vi "Execute Default event.vi"(4 "Module type":T1, 6 "Module ID":i32, 8 "error in":errorcluster, 9 "Event":string, 10 "DQMH Library Ref":refnum<vi>, 11 "application Instance":refnum<vi>) -> (0 "error out":errorcluster)   [LabVIEW 2019, in "Panther Dashboard.lvlib"]
doc: "This VI checks the Main.vi State of the selected DQMH Module"
uses:
  Panther Dashboard.lvlib
  Module type--enum.ctl
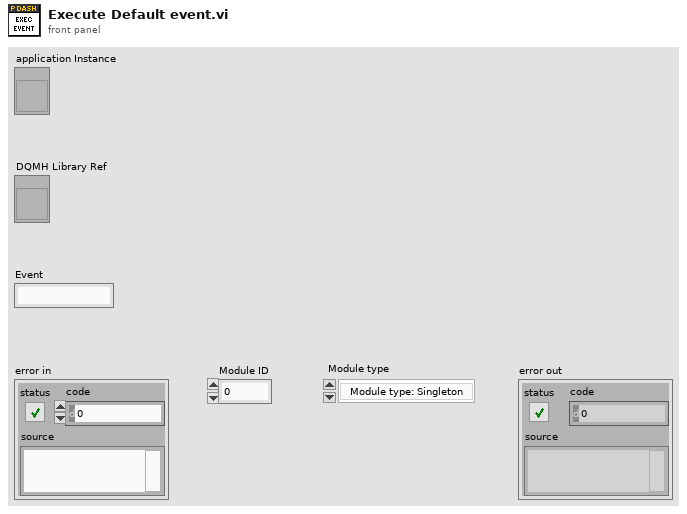
[diagram p1: front panel]
types:
  T1 = typedef "Panther Dashboard.lvlib/Module type--enum.ctl" = enum16{"Module type: Singleton", "Module type: Cloneable"}
  T2 = enum32{"Bad", "Idle", "Run top level", "Running"}
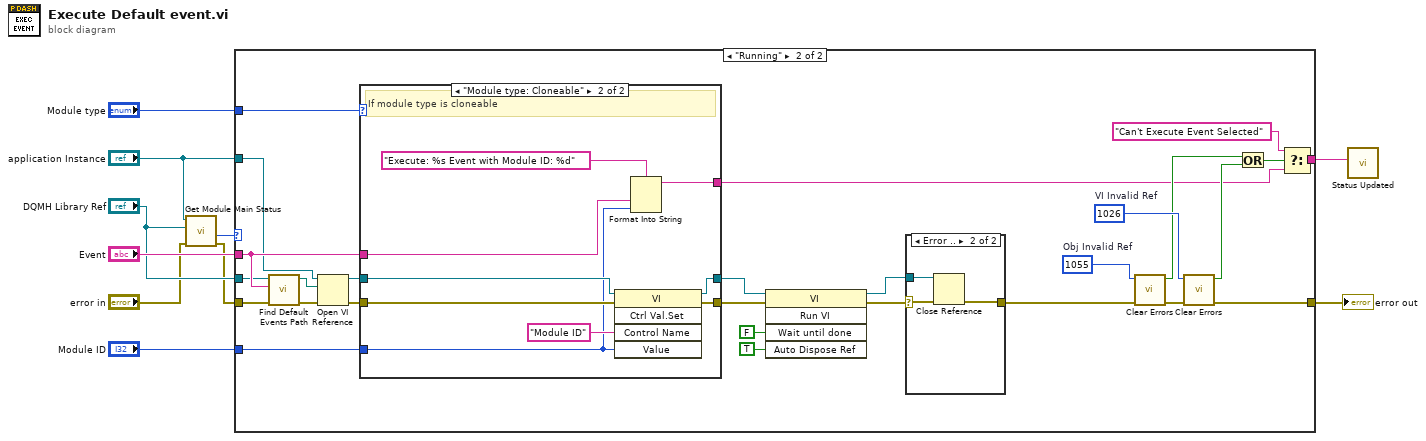
[diagram p0: block diagram]
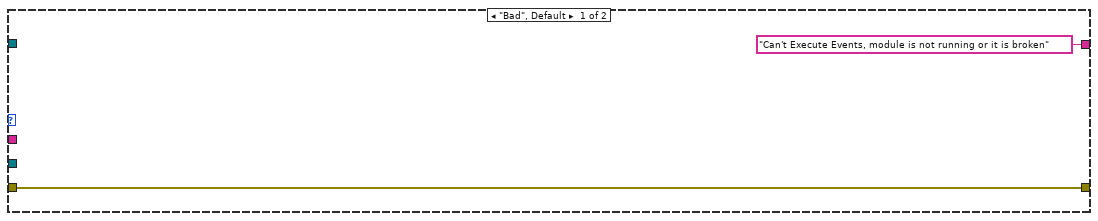
[diagram p2: hidden frame]
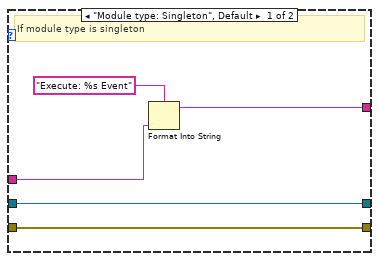
[diagram p4: hidden frame]
diagram:
  n1 = call "Get Module Main Status.vi"("error in"="error in", "Library in"="DQMH Library Ref", "application Instance"="application Instance") -> ("error out"=w1:errorcluster, "Module Exec State"=w3:T2)  [unwired: 6 in, 1 out]
  n2 = case shown="\"Running\"" w3 {
    tunnel: w1 -> [w12 w39]
    tunnel: [w12 w36] -> w10
    tunnel: "Module type" -> [_ w28]
    tunnel: "Module ID" -> [_ w26]
    tunnel: "Event" -> [_ w22]
    tunnel: ["Can't Execute Events, module is not running or it is broken" ("t") w17] -> w6
    tunnel: "application Instance" -> [_ w14]
    tunnel: "DQMH Library Ref" -> [_ w13]
    frame "Bad", Default {
    }
    frame "Running" {
      w30 = 1055  # Obj Invalid Ref
      w29 = 1026  # VI Invalid Ref
      n3 = call "Find Default Events Path.vi"("error in"=w39, "Event"=w22, "DQMH Library Ref"=w13) -> ("error out"=w38:errorcluster, "Event Path"=w31:path)  [unwired: 7 in]
      n4 = Open VI Reference(application reference (local)=w14, vi path=w31, error in (no error)=w38) -> (vi reference=w25:refnum<vi>, error out=w35:errorcluster)  [unwired: 3 in]
      n5 = case shown="\"Module type: Cloneable\"" w28 {
        tunnel: w25 -> [w47 w54]
        tunnel: w35 -> [w48 w56]
        tunnel: [w47 w53] -> w27
        tunnel: [w48 w57] -> w34
        tunnel: w26 -> [_ w51]
        tunnel: w22 -> [w45 w52]
        tunnel: [w44 w50] -> w18
        frame "Module type: Singleton", Default {
          # "If module type is singleton"
          n6 = Format Into String(format string="Execute: %s Event", w45) -> (resulting string=w44:string)  [unwired: 2 in, 1 out]
        }
        frame "Module type: Cloneable" {
          # "If module type is cloneable"
          n7 = invoke class="VI" method="Ctrl Val.Set"(reference=w54, error in=w56, "Control Name"="Module ID", "Value"=w51) -> (reference out=w53:refnum<vi>, error out=w57:errorcluster)  [unwired: 1 in, 3 out]
          n8 = Format Into String(format string="Execute: %s Event with Module ID: %d", w52, w51) -> (resulting string=w50:string)  [unwired: 2 in, 1 out]
        }
      }
      n9 = invoke class="VI" method="Run VI"(reference=w27, error in=w34, "Wait until done"=FALSE ("Wait Until Done"), "Auto Dispose Ref"=TRUE ("Auto Dispose Reference")) -> (reference out=w15:refnum<vi>, error out=w33:errorcluster)  [unwired: 1 in, 3 out]
      n10 = case shown="Error .." w33 {
        selector: w33 -> [w40 w42]
        tunnel: [w40 w43] -> w32
        tunnel: w15 -> [_ w41]
        frame No Error {
        }
        frame Error {
          n11 = Close Reference(reference=w41, error in (no error)=w42) -> (error out=w43:errorcluster)
        }
      }
      n12 = call <vilib>:"Clear Errors.vi"("error in (no error)"=w32, "specific error code to clear (0: all)"=w30) -> ("error out"=w37:errorcluster, "specific error cleared?"=w20:bool)  [unwired: 4 in]
      n13 = call <vilib>:"Clear Errors.vi"("error in (no error)"=w37, "specific error code to clear (0: all)"=w29) -> ("error out"=w36:errorcluster, "specific error cleared?"=w21:bool)  [unwired: 4 in]
      n14 = Or(x=w20, y=w21) -> (x .or. y?=w19:bool)
      n15 = Select(t="Can't Execute Event Selected", s=w19, f=w18) -> (s? t:f=w17:string)
    }
  }
  "error out" <- w10
  n16 = call "Status Updated.vi"("Status"=w6) -> ()  [unwired: 10 in, 1 out]
